vi "Auto_Step.vi"() -> ()   [LabVIEW 2020]
uses:
  Global_Variable/A180648.vi
  Global_Variable/Global.vi
panel:
  in  "判定结果":bool[][](array[boolean])=[[TRUE]]
  in  "VI引用句柄":refnum<vi>
  in  "前序OK？":string
  out "第三颗螺丝加力":bool
  out "第二颗螺丝加力":bool
  out "第一颗螺丝加力":bool
  out "磨合次数":i32
  in  "STEP":string
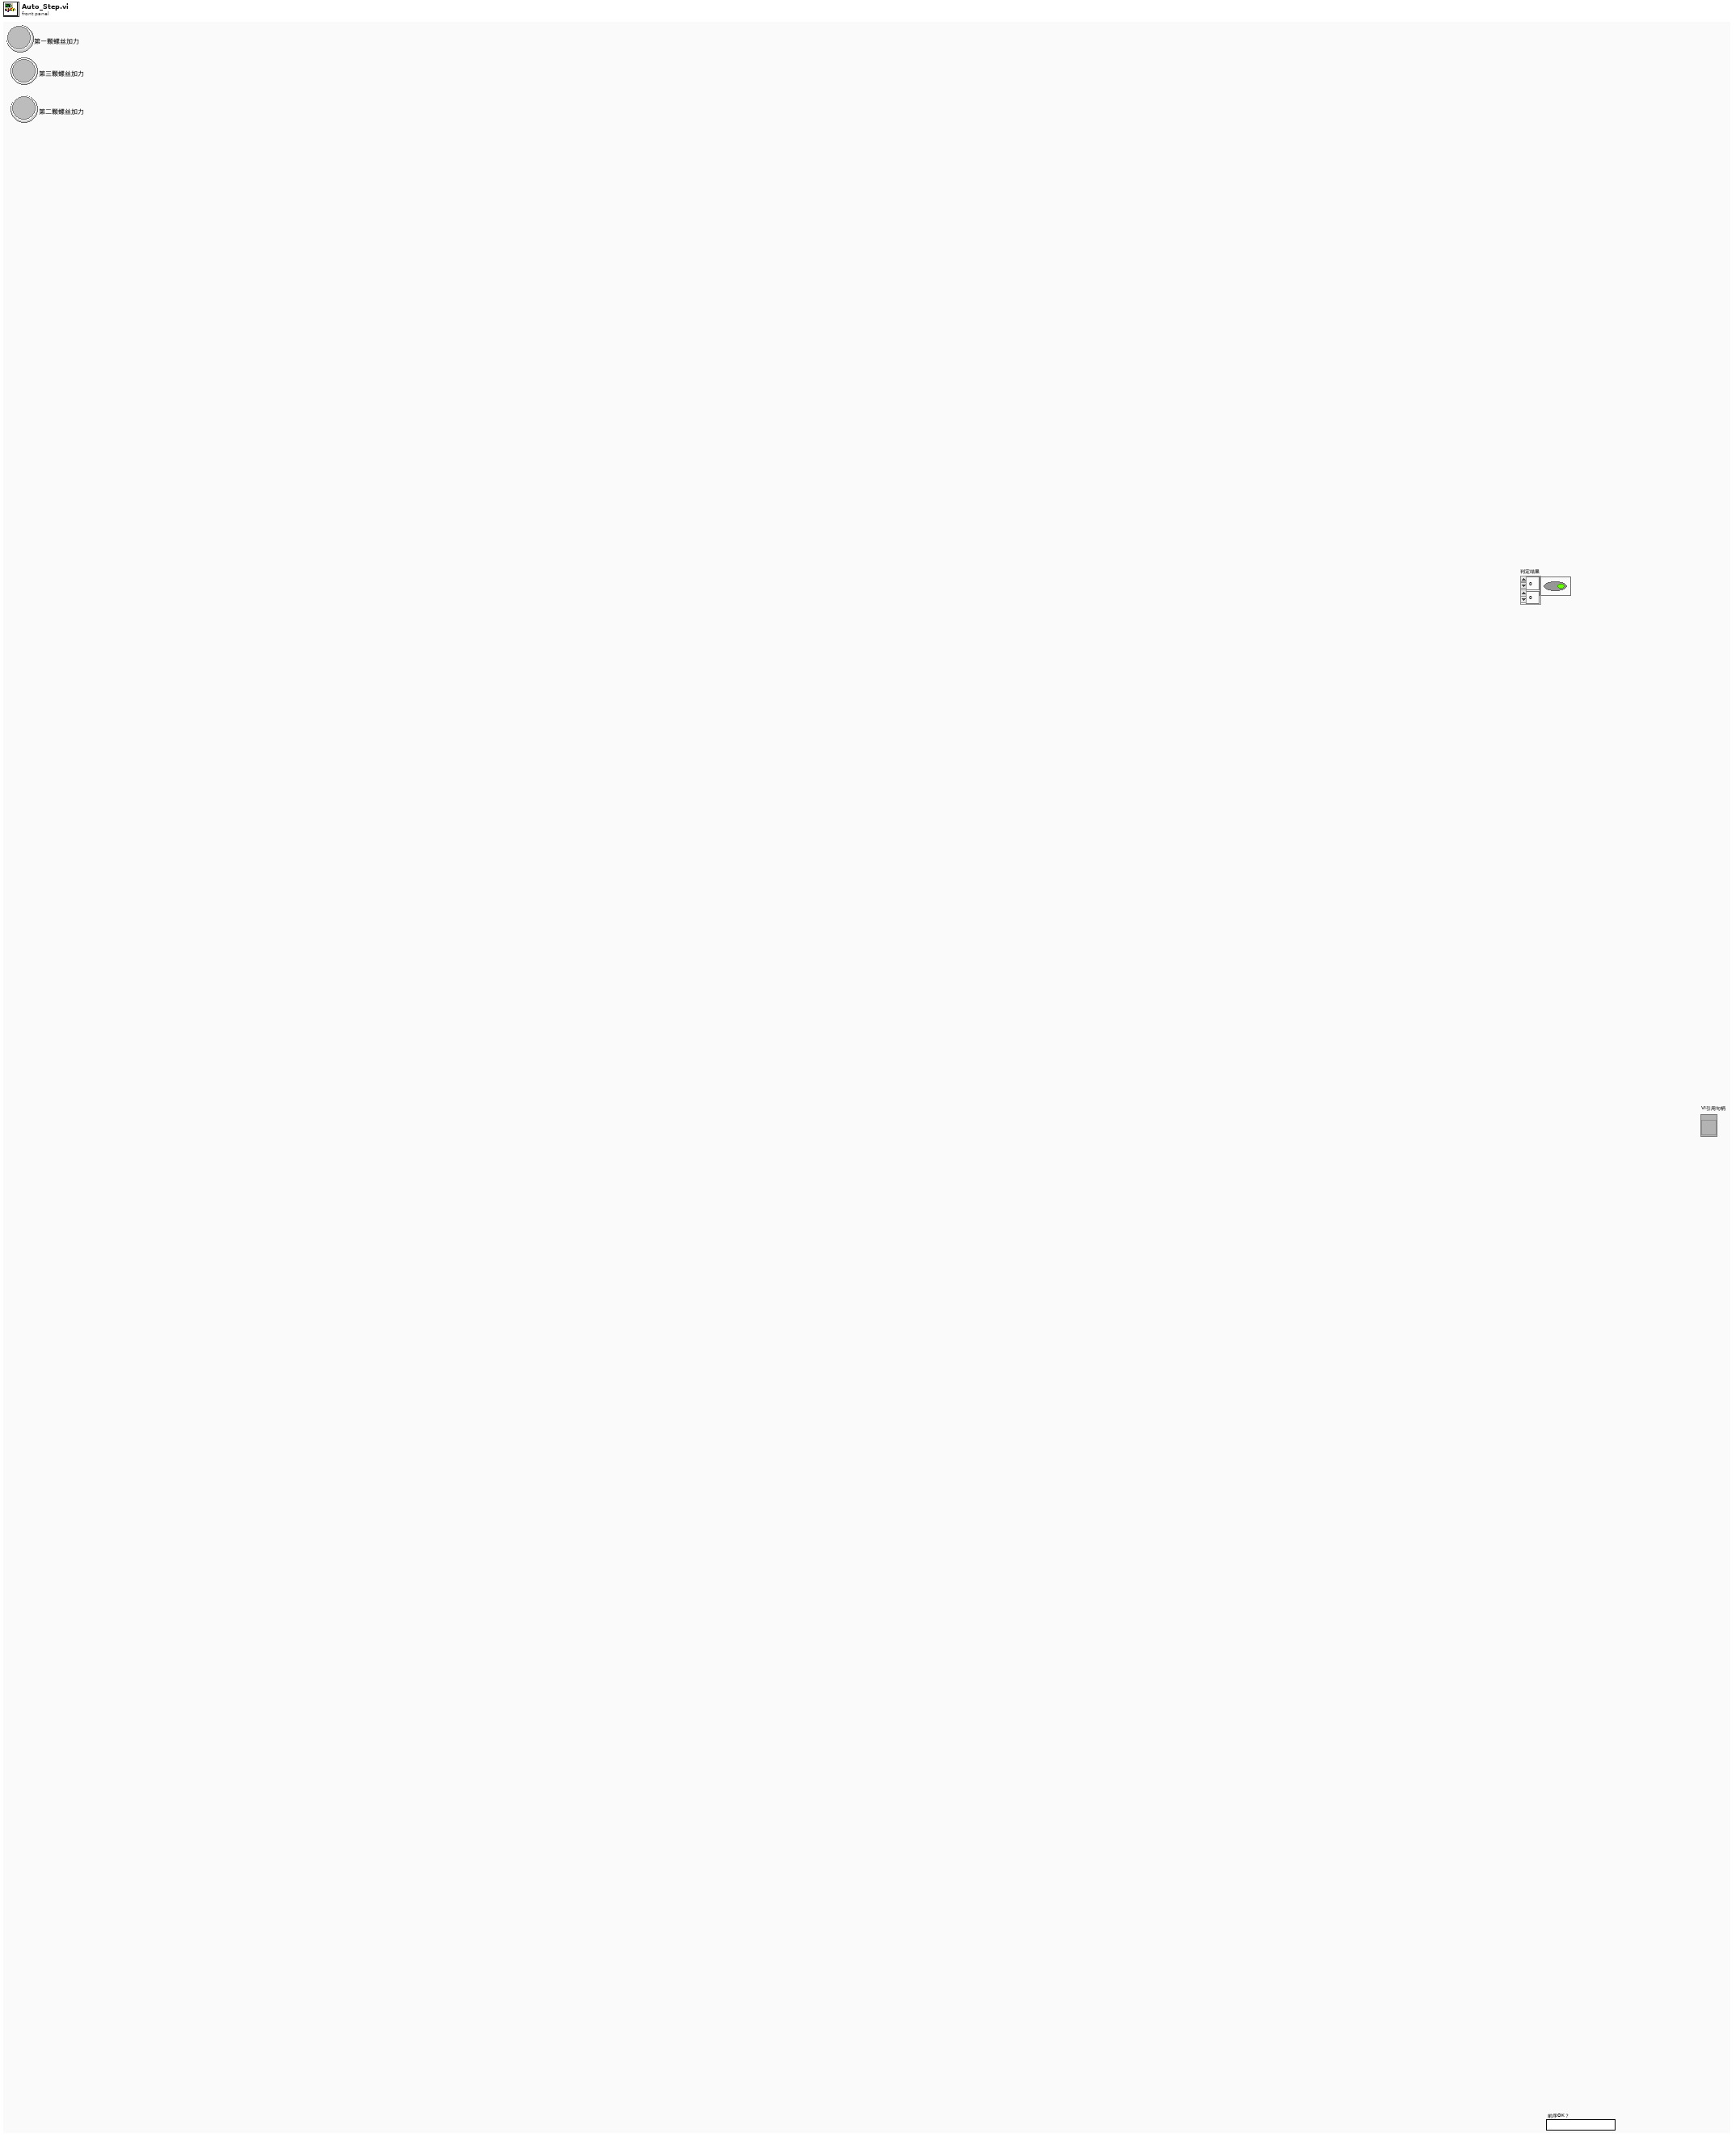
[diagram p1: front panel]
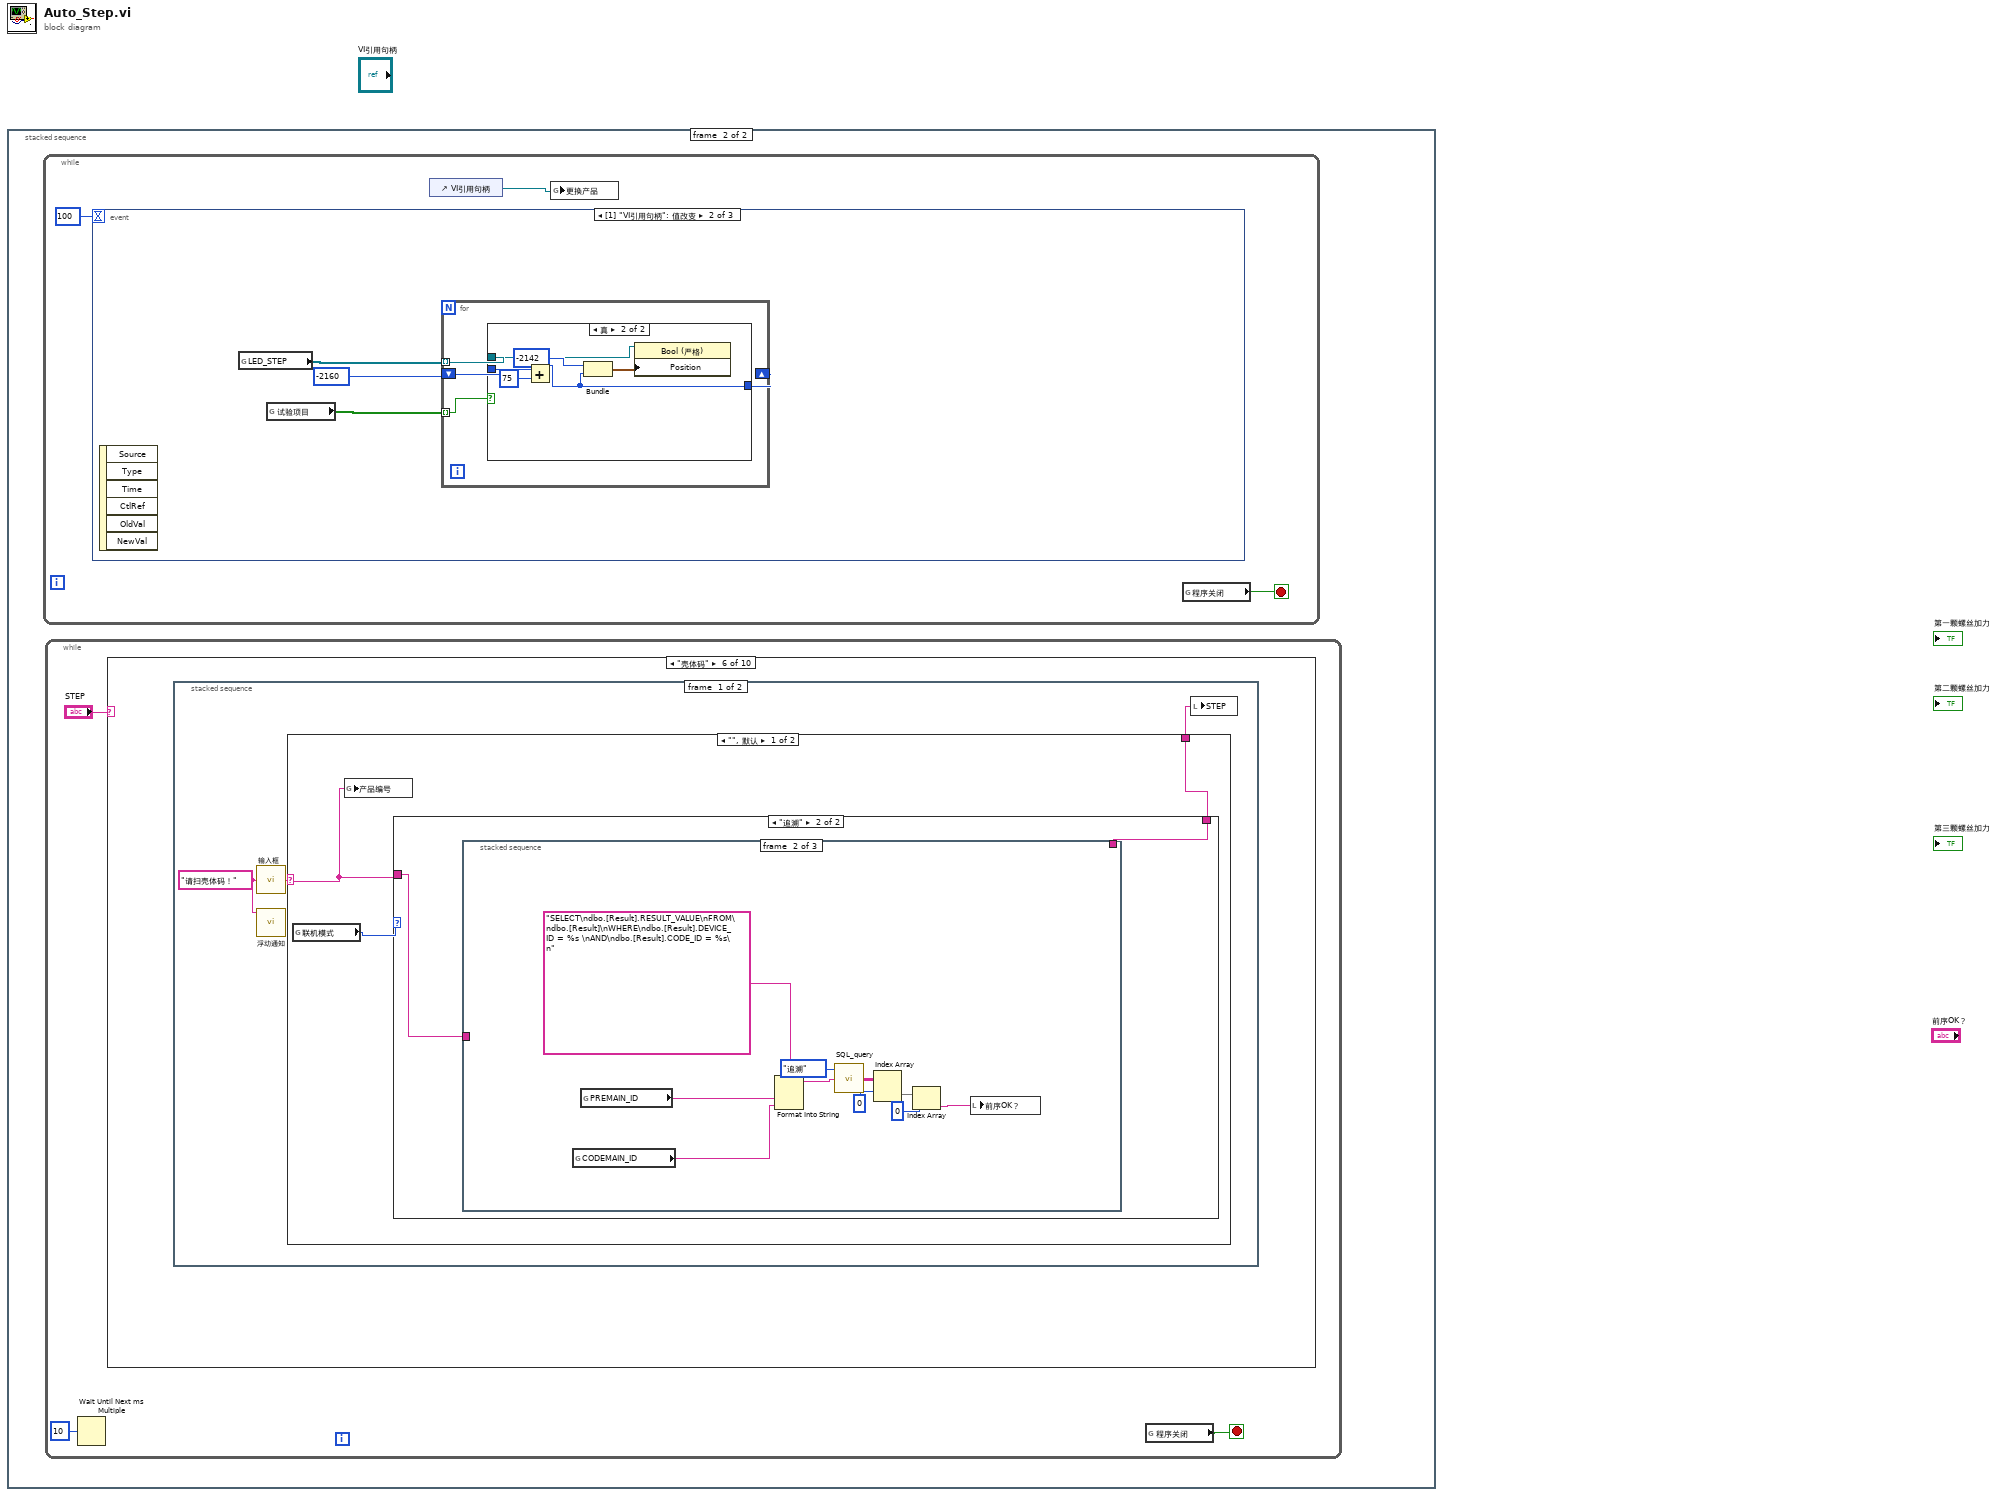
[diagram p0: block diagram]
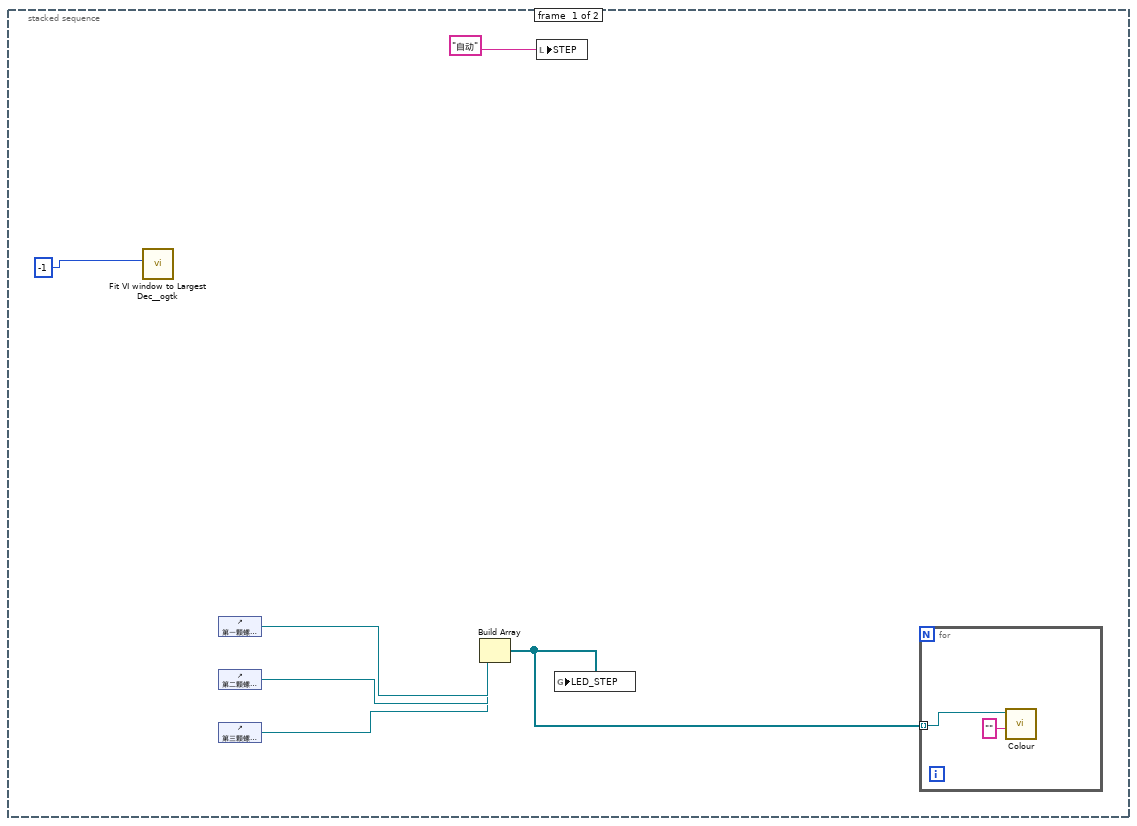
[diagram p2: hidden frame]
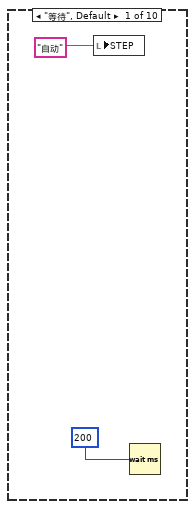
[diagram p3: hidden frame]
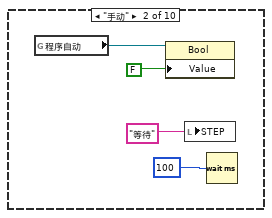
[diagram p4: hidden frame]
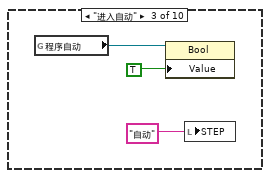
[diagram p5: hidden frame]
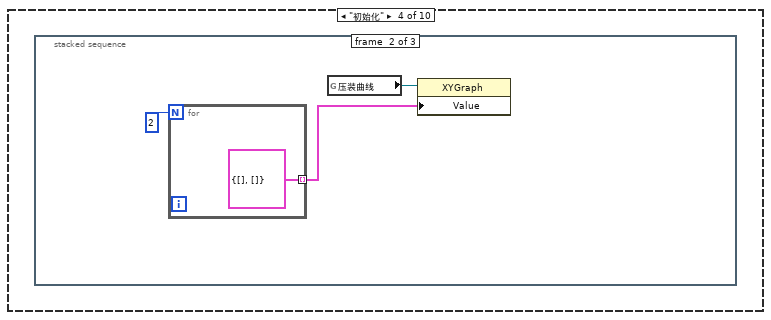
[diagram p6: hidden frame]
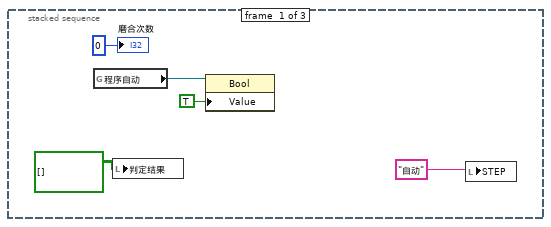
[diagram p7: hidden frame]
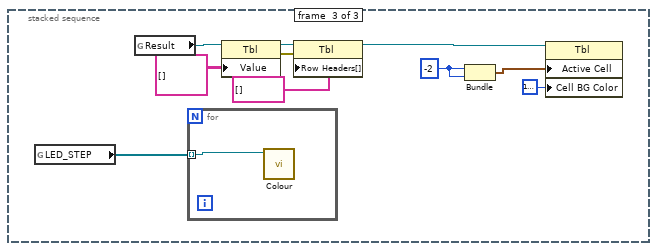
[diagram p8: hidden frame]
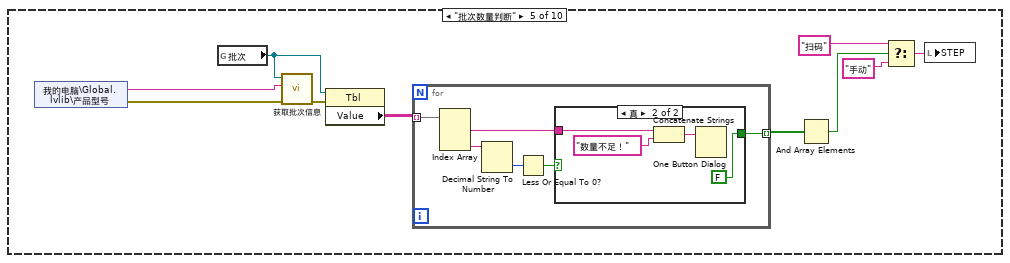
[diagram p9: hidden frame]
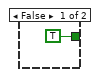
[diagram p10: hidden frame]
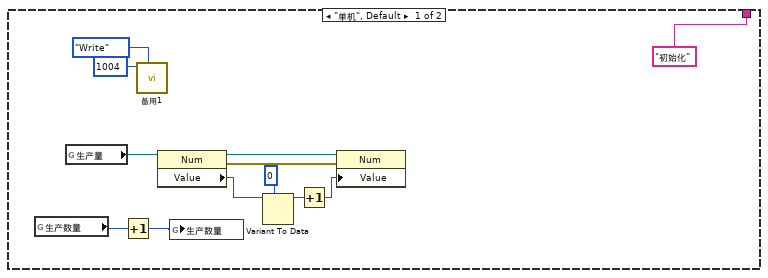
[diagram p11: hidden frame]
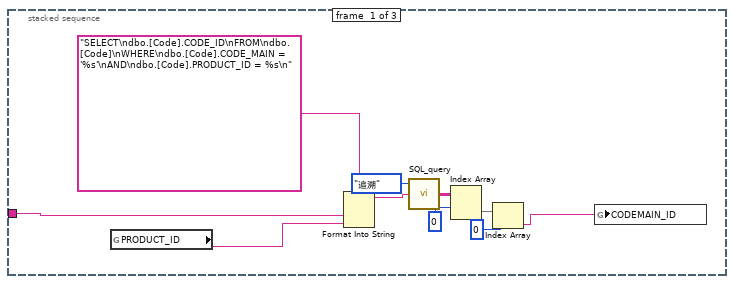
[diagram p12: hidden frame]
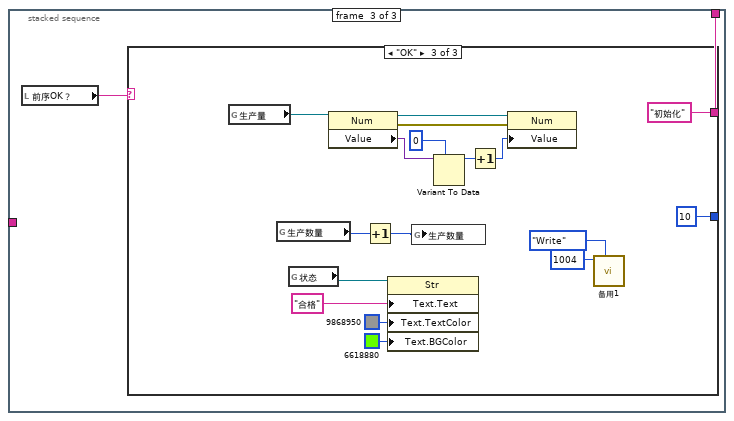
[diagram p13: hidden frame]
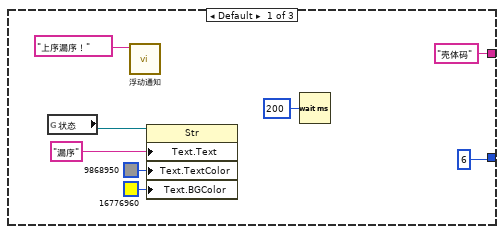
[diagram p14: hidden frame]
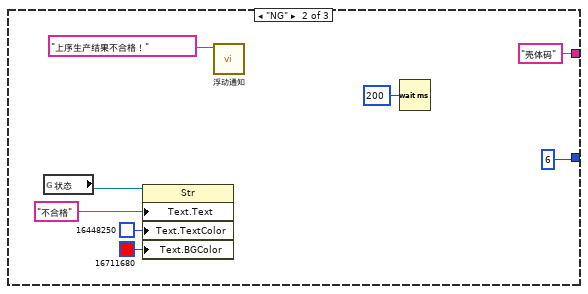
[diagram p15: hidden frame]
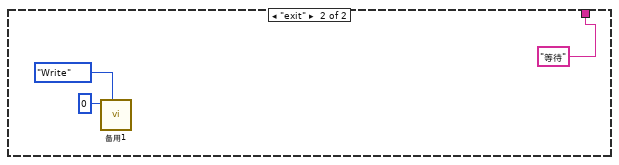
[diagram p16: hidden frame]
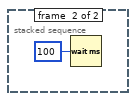
[diagram p17: hidden frame]
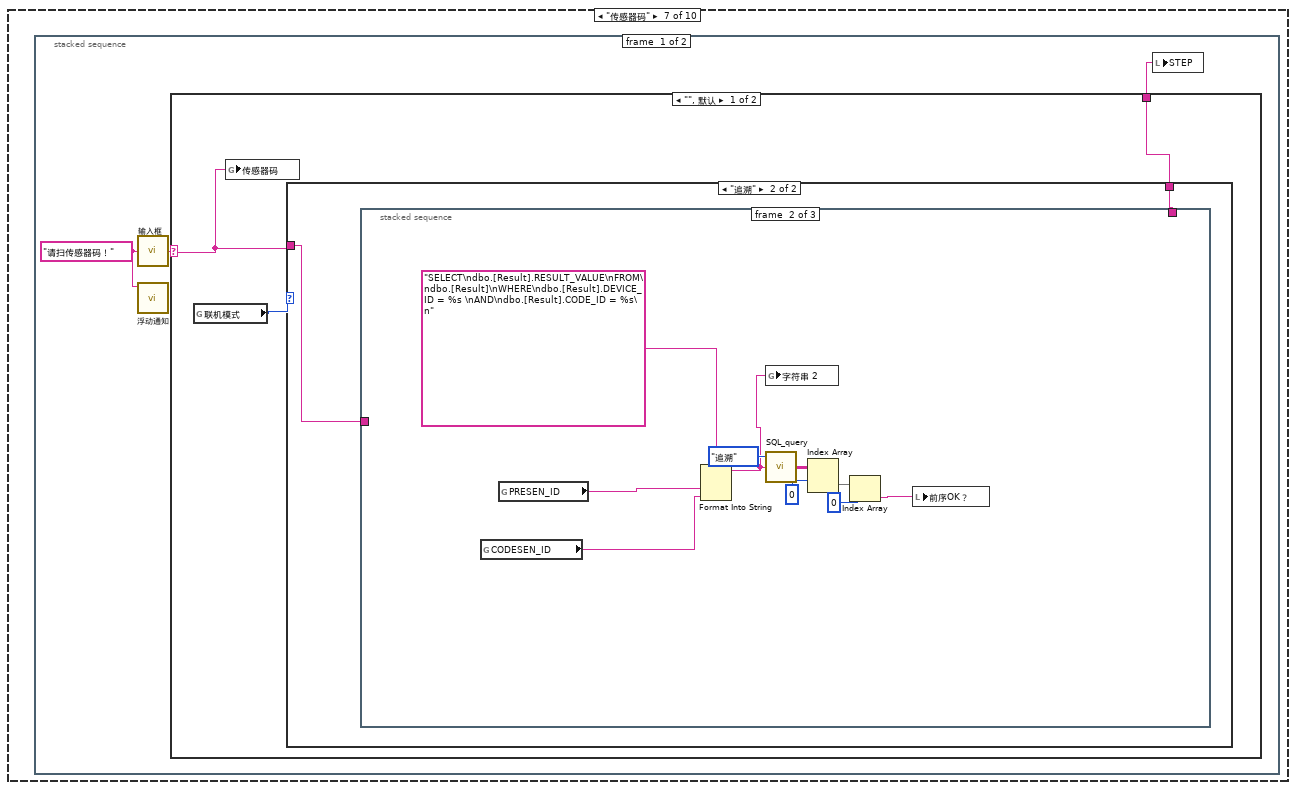
[diagram p18: hidden frame]
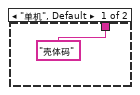
[diagram p19: hidden frame]
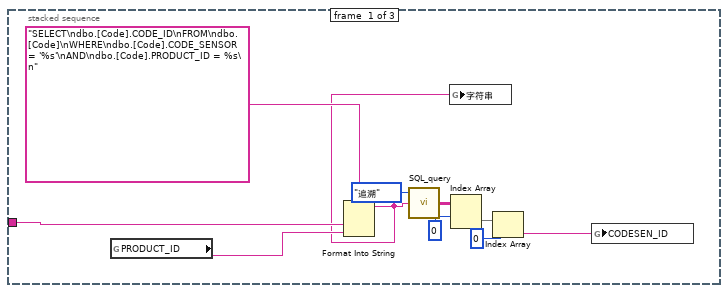
[diagram p20: hidden frame]
diagram:
  n1 = stacked-sequence {
    frame #0 {
      n2 = call <userlib>:"Fit VI window to Largest Dec__ogtk.vi"("border spacing (2 px)"=-1) -> ()  [unwired: 5 in, 2 out]
      n3 = control-ref of="第一颗螺丝加力"() -> (w4:refnum<vi>)
      n4 = control-ref of="第二颗螺丝加力"() -> (w3:refnum<vi>)
      n5 = control-ref of="第三颗螺丝加力"() -> (w2:refnum<vi>)
      n6 = Build Array(w4, w3, w2) -> (w1:refnum<vi>[])
      n7 = local write "STEP"("自动" ("STEP")) -> ()
      n8 = global write "A180648.vi" "LED_STEP"(w1) -> ()
      n9 = for {
        tunnel: w1 -> [w8] mode=indexing
        n10 = call "Colour.vi"("result"="", "colourRef"=w8) -> ()  [unwired: 9 in, 1 out]
      }
    }
    frame #1 {
      n11 = while {
        stop <- w324 stop-if-true
        n12 = event shown="[1] \"VI引用句柄\": 值改变" {
          selector: _ -> [_ _ _]
          dyn-events: _ -> [_ _ _]
          timeout: 100 -> [_ _ _]
          event Timeout {
            n13 = event-data() -> ()  [unwired: 1 in, 3 out]
          }
          event "VI引用句柄": Value Change {
            n14 = event-data() -> ()  [unwired: 1 in, 6 out]
            n15 = global read "A180648.vi" "LED_STEP"() -> (w326:refnum<vi>[])
            n16 = global read "Global.vi" "试验项目"() -> (w327:bool[])
            n17 = for "For循环" {
              tunnel: w327 -> [w329] mode=indexing
              tunnel: w326 -> [w332] mode=indexing
              shift-right: [w330] -> _
              shift-left: -2160 -> [w331]
              n18 = case shown="真" w329 {
                tunnel: w332 -> [w334 w336]
                tunnel: w331 -> [w335 w341]
                tunnel: [w335 w338] -> w330
                frame False {
                  n19 = property class="Bool (严格)"(reference=w334, "Top"=2000 ("位置:置顶")) -> ()  [unwired: 1 in, 2 out]
                }
                frame True {
                  n20 = Add(x=w341, y=75) -> (x+y=w338:i32)
                  n21 = Bundle(-2142, w338) -> (w339:cluster{i32, i32})  [unwired: 1 in]
                  n22 = property class="Bool (严格)"(reference=w336, "Position"=w339) -> ()  [unwired: 1 in, 2 out]
                }
              }
            }
          }
          event Panel Close {
            n23 = event-data() -> ()  [unwired: 1 in, 4 out]
            n24 = global write "Global.vi" "程序关闭"(TRUE ("程序关闭")) -> ()
          }
        }
        n25 = control-ref of="VI引用句柄"() -> (w323:refnum<vi>)
        n26 = global write "Global.vi" "更换产品"(w323) -> ()
        n27 = global read "Global.vi" "程序关闭"() -> (w324:bool)
      }
      n28 = while {
        stop <- w10 stop-if-true
        n29 = Wait Until Next ms Multiple(millisecond multiple=u32 10 ("毫秒倍数")) -> ()  [unwired: 1 out]
        n30 = case shown="\"壳体码\"" "STEP" {
          selector: "STEP" -> [_ _ _ _ _ _ _ w208 _ _]
          frame "等待", Default {
            n31 = local write "STEP"("自动" ("STEP")) -> ()
            n32 = Wait (ms)(milliseconds to wait=u32 200 ("等待时间（毫秒）")) -> ()  [unwired: 1 out]
          }
          frame "手动" {
            n33 = global read "Global.vi" "程序自动"() -> (w15:refnum<vi>)
            n34 = property class="Bool"(reference=w15, "Value"=FALSE) -> ()  [unwired: 1 in, 2 out]
            n35 = local write "STEP"("等待" ("STEP")) -> ()
            n36 = Wait (ms)(milliseconds to wait=u32 100 ("等待时间（毫秒）")) -> ()  [unwired: 1 out]
          }
          frame "进入自动" {
            n37 = global read "Global.vi" "程序自动"() -> (w19:refnum<vi>)
            n38 = property class="Bool"(reference=w19, "Value"=TRUE) -> ()  [unwired: 1 in, 2 out]
            n39 = local write "STEP"("自动" ("STEP")) -> ()
          }
          frame "初始化" {
            n40 = stacked-sequence {
              frame #0 {
                n41 = global read "Global.vi" "程序自动"() -> (w24:refnum<vi>)
                n42 = local write "判定结果"(bool[][] [] ("判定结果")) -> ()
                n43 = property class="Bool"(reference=w24, "Value"=TRUE) -> ()  [unwired: 1 in, 2 out]
                n44 = local write "STEP"("自动" ("result")) -> ()
                "磨合次数" <- 0 ("磨合次数")
              }
              frame #1 {
                n45 = for {
                  N: 2 -> [_]
                  tunnel: [cluster{dbl[], dbl[]} {[], []}] -> w26 mode=indexing
                }
                n46 = global read "A180648.vi" "压装曲线"() -> (w27:refnum<vi>)
                n47 = property class="XYGraph"(reference=w27, "Value"=w26) -> ()  [unwired: 1 in, 2 out]
              }
              frame #2 {
                w33 = -2
                n48 = global read "A180648.vi" "LED_STEP"() -> (w30:refnum<vi>[])
                n49 = global read "Global.vi" "Result"() -> (w37:refnum<vi>)
                n50 = for {
                  tunnel: w30 -> [w40] mode=indexing
                  n51 = call "Colour.vi"("colourRef"=w40) -> ()  [unwired: 10 in, 1 out]
                }
                n52 = property class="Tbl"(reference=w37, "Value"=string[][] []) -> (reference out=w38:refnum<vi>, error out=w39:errorcluster)  [unwired: 1 in]
                n53 = property class="Tbl"(reference=w38, error in=w39, "Row Headers[]"=string[] [] ("行首字符串[]")) -> (reference out=w34:refnum<vi>)  [unwired: 1 out]
                n54 = Bundle(w33, w33) -> (w32:cluster{i32, i32})  [unwired: 1 in]
                n55 = property class="Tbl"(reference=w34, "Active Cell"=w32, "Cell BG Color"=u32 16777216 ("活动单元格:单元格背景色")) -> ()  [unwired: 1 in, 2 out]
              }
            }
          }
          frame "批次数量判断" {
            n56 = shared-variable "我的电脑\\Global.lvlib\\产品型号"() -> (w46:string, error out=w49:errorcluster)  [unwired: 1 in]
            n57 = global read "Global.vi" "批次"() -> (w47:refnum<vi>)
            n58 = call "获取批次信息.vi"("error in (no error)"=w49, "产品型号"=w46, "Tbl引用句柄"=w47) -> ("error out"=w48:errorcluster)  [unwired: 7 in, 1 out]
            n59 = property class="Tbl"(reference=w47, error in=w48) -> ("Value"=w50:string[][])  [unwired: 2 out]
            n60 = for {
              tunnel: w50 -> [w56] mode=indexing
              tunnel: [w51] -> w45 mode=indexing
              n61 = Index Array(array=w56) -> (element #1=w52:string, element #3=w55:string)  [unwired: 3 in, 1 out]
              n62 = Decimal String To Number(string=w55) -> (number=w54:i32)  [unwired: 2 in, 1 out]
              n63 = Less Or Equal To 0?(x=w54) -> (x <= 0?=w53:bool)
              n64 = case shown="真" w53 {
                tunnel: w52 -> [_ w61]
                tunnel: [TRUE FALSE] -> w51
                frame False {
                }
                frame True {
                  n65 = Concatenate Strings(w61, "数量不足！" ("字符串")) -> (w59:string)
                  n66 = One Button Dialog(message=w59) -> ()  [unwired: 1 in, 1 out]
                }
              }
            }
            n67 = And Array Elements(Boolean array=w45) -> (logical AND=w44:bool)
            n68 = Select(t="扫码" ("STEP"), s=w44, f="手动" ("STEP")) -> (s? t:f=w41:string)
            n69 = local write "STEP"(w41) -> ()
          }
          frame "壳体码" {
            n70 = stacked-sequence {
              frame #0 {
                w63 = "请扫壳体码！" ("提示信息")
                n71 = call "输入框.vi"("提示信息"=w63) -> ("条形码输出"=w64:string)
                n72 = call "浮动通知.vi"("通知内容"=w63) -> ()  [unwired: 11 in]
                n73 = case shown="\"\", 默认" w64 {
                  selector: w64 -> [w65 _]
                  tunnel: [w67 "等待"] -> w62
                  frame "", Default {
                    n74 = global read "Global.vi" "联机模式"() -> (w66:enum16{"单机", "追溯"})
                    n75 = global write "Global.vi" "产品编号"(w65) -> ()
                    n76 = case shown="\"追溯\"" w66 {
                      tunnel: w65 -> [_ w80]
                      tunnel: ["初始化" w81] -> w67
                      frame "单机", Default {
                        n77 = global read "Global.vi" "生产数量"() -> (w69:i32)
                        n78 = global read "Global.vi" "生产量"() -> (w72:refnum<vi>)
                        n79 = Increment(x=w69) -> (x+1=w68:i32)
                        n80 = call "备用1.vi"("枚举"=enum16{"Read", "Write"}."Write", "Status_Write"=i16 1004) -> ()  [unwired: 9 in, 1 out]
                        n81 = property class="Num"(reference=w72) -> (reference out=w75:refnum<vi>, error out=w76:errorcluster, "Value"=w77:variant)  [unwired: 1 in]
                        n82 = global write "Global.vi" "生产数量"(w68) -> ()
                        n83 = Variant To Data(type=u32 0, Variant=w77) -> (data=w78:u32)  [unwired: 1 in, 1 out]
                        n84 = Increment(x=w78) -> (x+1=w79:u32)
                        n85 = property class="Num"(reference=w75, error in=w76, "Value"=w79) -> ()  [unwired: 2 out]
                      }
                      frame "追溯" {
                        n86 = stacked-sequence {
                          tunnel: w80 -> [w89 _ _]
                          tunnel: [_ _ w103] -> w81
                          frame #0 {
                            n87 = global read "追溯Global.vi" "PRODUCT_ID"() -> (w83:string)
                            n88 = Format Into String(format string="SELECT\ndbo.[Code].CODE_ID\nFROM\ndbo.[Code]\nWHERE\ndbo.[Code].CODE_MAIN = '%s'\nAND\ndbo.[Code].PRODUCT_ID = %s\n" ("格式字符串"), w89, w83) -> (resulting string=w88:string)  [unwired: 2 in, 1 out]
                            n89 = call "SQL_query.vi"("SQL query"=w88, "联机模式"=enum16{"单机", "追溯"}."追溯") -> ("data"=w91:string[][])  [unwired: 2 in, 1 out]
                            n90 = Index Array(array=w91, index (row)=0 ("索引 (行)")) -> (element=w90:string[])  [unwired: 1 in]
                            n91 = Index Array(array=w90, index=0 ("索引")) -> (element=w84:string)
                            n92 = global write "追溯Global.vi" "CODEMAIN_ID"(w84) -> ()
                          }
                          frame #1 {
                            n93 = global read "追溯Global.vi" "CODEMAIN_ID"() -> (w92:string)
                            n94 = global read "追溯Global.vi" "PREMAIN_ID"() -> (w94:string)
                            n95 = Format Into String(format string="SELECT\ndbo.[Result].RESULT_VALUE\nFROM\ndbo.[Result]\nWHERE\ndbo.[Result].DEVICE_ID = %s \nAND\ndbo.[Result].CODE_ID = %s\n" ("格式字符串"), w94, w92) -> (resulting string=w99:string)  [unwired: 2 in, 1 out]
                            n96 = call "SQL_query.vi"("SQL query"=w99, "联机模式"=enum16{"单机", "追溯"}."追溯") -> ("data"=w101:string[][])  [unwired: 2 in, 1 out]
                            n97 = Index Array(array=w101, index (row)=0 ("索引 (行)")) -> (element=w100:string[])  [unwired: 1 in]
                            n98 = Index Array(array=w100, index=0 ("索引")) -> (element=w95:string)
                            n99 = local write "前序OK？"(w95) -> ()
                          }
                          frame #2 {
                            n100 = local read "前序OK？"() -> (w102:string)
                            n101 = case shown="\"OK\"" w102 {
                              tunnel: [i16 6 ("设备状态控制字") i16 6 ("设备状态控制字") i16 10 ("设备状态控制字")] -> _
                              tunnel: ["壳体码" "壳体码" "初始化"] -> w103
                              frame Default {
                                n102 = global read "Global.vi" "状态"() -> (w107:refnum<vi>)
                                n103 = call "浮动通知.vi"("通知内容"="上序漏序！" ("Status")) -> ()  [unwired: 11 in]
                                n104 = property class="Str"(reference=w107, "Text.Text"="漏序" ("文本.文本"), "Text.TextColor"=u32 9868950 ("文本.文本颜色:文本颜色"), "Text.BGColor"=u32 16776960 ("文本.文本颜色:背景色")) -> ()  [unwired: 1 in, 2 out]
                                n105 = Wait (ms)(milliseconds to wait=u32 200 ("等待时间（毫秒）")) -> ()  [unwired: 1 out]
                              }
                              frame "NG" {
                                n106 = global read "Global.vi" "状态"() -> (w115:refnum<vi>)
                                n107 = property class="Str"(reference=w115, "Text.Text"="不合格" ("文本.文本"), "Text.TextColor"=u32 16448250 ("文本.文本颜色:文本颜色"), "Text.BGColor"=u32 16711680 ("文本.文本颜色:背景色")) -> ()  [unwired: 1 in, 2 out]
                                n108 = call "浮动通知.vi"("通知内容"="上序生产结果不合格！" ("Status")) -> ()  [unwired: 11 in]
                                n109 = Wait (ms)(milliseconds to wait=u32 200 ("等待时间（毫秒）")) -> ()  [unwired: 1 out]
                              }
                              frame "OK" {
                                n110 = global read "Global.vi" "生产量"() -> (w128:refnum<vi>)
                                n111 = global read "Global.vi" "生产数量"() -> (w123:i32)
                                n112 = global read "Global.vi" "状态"() -> (w127:refnum<vi>)
                                n113 = property class="Num"(reference=w128) -> (reference out=w135:refnum<vi>, error out=w134:errorcluster, "Value"=w133:variant)  [unwired: 1 in]
                                n114 = Increment(x=w123) -> (x+1=w122:i32)
                                n115 = property class="Str"(reference=w127, "Text.Text"="合格" ("文本.文本"), "Text.TextColor"=u32 9868950 ("文本.文本颜色:文本颜色"), "Text.BGColor"=u32 6618880 ("文本.文本颜色:背景色")) -> ()  [unwired: 1 in, 2 out]
                                n116 = global write "Global.vi" "生产数量"(w122) -> ()
                                n117 = Variant To Data(type=u32 0, Variant=w133) -> (data=w132:u32)  [unwired: 1 in, 1 out]
                                n118 = Increment(x=w132) -> (x+1=w131:u32)
                                n119 = property class="Num"(reference=w135, error in=w134, "Value"=w131) -> ()  [unwired: 2 out]
                                n120 = call "备用1.vi"("枚举"=enum16{"Read", "Write"}."Write", "Status_Write"=i16 1004) -> ()  [unwired: 9 in, 1 out]
                              }
                            }
                          }
                        }
                      }
                    }
                  }
                  frame "exit" {
                    n121 = call "备用1.vi"("枚举"=enum16{"Read", "Write"}."Write", "Status_Write"=i16 0) -> ()  [unwired: 9 in, 1 out]
                  }
                }
                n122 = local write "STEP"(w62) -> ()
              }
              frame #1 {
                n123 = Wait (ms)(milliseconds to wait=u32 100 ("等待时间（毫秒）")) -> ()  [unwired: 1 out]
              }
            }
          }
          frame "传感器码" {
            n124 = stacked-sequence {
              frame #0 {
                w142 = "请扫传感器码！" ("提示信息")
                n125 = call "输入框.vi"("提示信息"=w142) -> ("条形码输出"=w143:string)
                n126 = call "浮动通知.vi"("通知内容"=w142) -> ()  [unwired: 11 in]
                n127 = case shown="\"\", 默认" w143 {
                  selector: w143 -> [w144 _]
                  tunnel: [w146 "等待"] -> w141
                  frame "", Default {
                    n128 = global read "Global.vi" "联机模式"() -> (w145:enum16{"单机", "追溯"})
                    n129 = global write "Global.vi" "传感器码"(w144) -> ()
                    n130 = case shown="\"追溯\"" w145 {
                      tunnel: w144 -> [_ w148]
                      tunnel: ["壳体码" w149] -> w146
                      frame "单机", Default {
                      }
                      frame "追溯" {
                        n131 = stacked-sequence {
                          tunnel: w148 -> [w157 _ _]
                          tunnel: [_ _ w171] -> w149
                          frame #0 {
                            n132 = global read "追溯Global.vi" "PRODUCT_ID"() -> (w152:string)
                            n133 = Format Into String(format string="SELECT\ndbo.[Code].CODE_ID\nFROM\ndbo.[Code]\nWHERE\ndbo.[Code].CODE_SENSOR = '%s'\nAND\ndbo.[Code].PRODUCT_ID = %s\n" ("格式字符串"), w157, w152) -> (resulting string=w150:string)  [unwired: 2 in, 1 out]
                            n134 = call "SQL_query.vi"("SQL query"=w150, "联机模式"=enum16{"单机", "追溯"}."追溯") -> ("data"=w159:string[][])  [unwired: 2 in, 1 out]
                            n135 = global write "追溯Global.vi" "字符串"(w150) -> ()
                            n136 = Index Array(array=w159, index (row)=0 ("索引 (行)")) -> (element=w158:string[])  [unwired: 1 in]
                            n137 = Index Array(array=w158, index=0 ("索引")) -> (element=w153:string)
                            n138 = global write "追溯Global.vi" "CODESEN_ID"(w153) -> ()
                          }
                          frame #1 {
                            n139 = global read "追溯Global.vi" "CODESEN_ID"() -> (w160:string)
                            n140 = global read "追溯Global.vi" "PRESEN_ID"() -> (w162:string)
                            n141 = Format Into String(format string="SELECT\ndbo.[Result].RESULT_VALUE\nFROM\ndbo.[Result]\nWHERE\ndbo.[Result].DEVICE_ID = %s \nAND\ndbo.[Result].CODE_ID = %s\n" ("格式字符串"), w162, w160) -> (resulting string=w161:string)  [unwired: 2 in, 1 out]
                            n142 = global write "追溯Global.vi" "字符串 2"(w161) -> ()
                            n143 = call "SQL_query.vi"("SQL query"=w161, "联机模式"=enum16{"单机", "追溯"}."追溯") -> ("data"=w169:string[][])  [unwired: 2 in, 1 out]
                            n144 = Index Array(array=w169, index (row)=0 ("索引 (行)")) -> (element=w168:string[])  [unwired: 1 in]
                            n145 = Index Array(array=w168, index=0 ("索引")) -> (element=w164:string)
                            n146 = local write "前序OK？"(w164) -> ()
                          }
                          frame #2 {
                            n147 = local read "前序OK？"() -> (w170:string)
                            n148 = case shown="\"NG\"" w170 {
                              tunnel: [i16 6 ("设备状态控制字") i16 6 ("设备状态控制字") i16 10 ("设备状态控制字")] -> _
                              tunnel: ["传感器码" "传感器码" "壳体码"] -> w171
                              frame Default {
                                n149 = global read "Global.vi" "状态"() -> (w175:refnum<vi>)
                                n150 = property class="Str"(reference=w175, "Text.Text"="漏序" ("文本.文本"), "Text.TextColor"=u32 9868950 ("文本.文本颜色:文本颜色"), "Text.BGColor"=u32 16776960 ("文本.文本颜色:背景色")) -> ()  [unwired: 1 in, 2 out]
                                n151 = call "浮动通知.vi"("通知内容"="上序漏序！" ("Status")) -> ()  [unwired: 11 in]
                                n152 = Wait (ms)(milliseconds to wait=u32 200 ("等待时间（毫秒）")) -> ()  [unwired: 1 out]
                              }
                              frame "NG" {
                                n153 = global read "Global.vi" "状态"() -> (w183:refnum<vi>)
                                n154 = property class="Str"(reference=w183, "Text.Text"="不合格" ("文本.文本"), "Text.TextColor"=u32 16448250 ("文本.文本颜色:文本颜色"), "Text.BGColor"=u32 16711680 ("文本.文本颜色:背景色")) -> ()  [unwired: 1 in, 2 out]
                                n155 = call "浮动通知.vi"("通知内容"="上序生产结果不合格！" ("Status")) -> ()  [unwired: 11 in]
                                n156 = Wait (ms)(milliseconds to wait=u32 200 ("等待时间（毫秒）")) -> ()  [unwired: 1 out]
                              }
                              frame "OK" {
                                n157 = global read "Global.vi" "生产量"() -> (w192:refnum<vi>)
                                n158 = global read "Global.vi" "状态"() -> (w191:refnum<vi>)
                                n159 = property class="Num"(reference=w192) -> (reference out=w199:refnum<vi>, error out=w198:errorcluster, "Value"=w197:variant)  [unwired: 1 in]
                                n160 = property class="Str"(reference=w191, "Text.Text"="合格" ("文本.文本"), "Text.TextColor"=u32 9868950 ("文本.文本颜色:文本颜色"), "Text.BGColor"=u32 6618880 ("文本.文本颜色:背景色")) -> ()  [unwired: 1 in, 2 out]
                                n161 = Variant To Data(type=u32 0, Variant=w197) -> (data=w196:u32)  [unwired: 1 in, 1 out]
                                n162 = Increment(x=w196) -> (x+1=w195:u32)
                                n163 = property class="Num"(reference=w199, error in=w198, "Value"=w195) -> ()  [unwired: 2 out]
                              }
                            }
                          }
                        }
                      }
                    }
                  }
                  frame "exit" {
                    n164 = call "备用1.vi"("枚举"=enum16{"Read", "Write"}."Write", "Status_Write"=i16 0) -> ()  [unwired: 9 in, 1 out]
                  }
                }
                n165 = local write "STEP"(w141) -> ()
              }
              frame #1 {
                n166 = Wait (ms)(milliseconds to wait=u32 100 ("等待时间（毫秒）")) -> ()  [unwired: 1 out]
              }
            }
          }
          frame "自动" {
            n167 = global read "A180648.vi" "LED_STEP"() -> (w207:refnum<vi>[])
            n168 = global read "Global.vi" "设备状态"() -> (w206:i16)
            n169 = case shown="71" w206 {
              tunnel: w207 -> [_ _ _ w217 w223 w230 w235 w236 _ _ _ w239 w243 w248 w253 w258 w264 _ w269 _ _ _ _]
              tunnel: w208 -> [_ _ _ _ _ _ _ _ _ _ _ _ _ _ _ _ _ _ _ _ _ _ _]
              frame Default {
              }
              frame -128 {
                n170 = call "浮动通知.vi"("通知内容"="复位中……" ("Status")) -> ()  [unwired: 11 in]
                n171 = global read "Global.vi" "程序自动"() -> (w212:refnum<vi>)
                n172 = property class="Bool"(reference=w212, "Value"=FALSE) -> ()  [unwired: 1 in, 2 out]
              }
              frame 0 {
              }
              frame 2 {
                n173 = Index Array(array=w217) -> (element=w216:refnum<vi>)  [unwired: 1 in]
                n174 = call "浮动通知.vi"("通知内容"="请拧紧第一颗螺丝" ("Status")) -> ()  [unwired: 11 in]
                n175 = call "Colour.vi"("result"="等待", "colourRef"=w216) -> ()  [unwired: 9 in, 1 out]
              }
              frame 3 {
                n176 = Index Array(array=w223) -> (element #1=w222:refnum<vi>, element #2=w218:refnum<vi>)  [unwired: 2 in]
                n177 = call "浮动通知.vi"("通知内容"="请拧紧第二颗螺丝" ("Status")) -> ()  [unwired: 11 in]
                n178 = call "Colour.vi"("result"="等待", "colourRef"=w218) -> ()  [unwired: 9 in, 1 out]
                n179 = call "Colour.vi"("result"="OK", "colourRef"=w222) -> ()  [unwired: 9 in, 1 out]
              }
              frame 4 {
                n180 = Index Array(array=w230, index #1=1 ("索引")) -> (element #1=w229:refnum<vi>, element #2=w225:refnum<vi>)  [unwired: 1 in]
                n181 = call "浮动通知.vi"("通知内容"="请拧紧第三颗螺丝" ("Status")) -> ()  [unwired: 11 in]
                n182 = call "Colour.vi"("result"="等待", "colourRef"=w225) -> ()  [unwired: 9 in, 1 out]
                n183 = call "Colour.vi"("result"="OK", "colourRef"=w229) -> ()  [unwired: 9 in, 1 out]
              }
              frame 5 {
                n184 = Index Array(array=w235, index #1=2 ("索引")) -> (element #1=w234:refnum<vi>)  [unwired: 1 in, 1 out]
                n185 = call "浮动通知.vi"("通知内容"="请标记" ("Status")) -> ()  [unwired: 11 in]
                n186 = call "Colour.vi"("result"="OK", "colourRef"=w234) -> ()  [unwired: 9 in, 1 out]
              }
              frame 6 {
                n187 = Index Array(array=w236, index=0 ("索引")) -> ()  [unwired: 1 out]
              }
              frame 7 {
              }
              frame 8 {
              }
              frame 9 {
              }
              frame 10 {
                n188 = Index Array(array=w239, index #1=0 ("索引")) -> ()  [unwired: 1 in, 2 out]
                n189 = call "Colour.vi"("result"="OK") -> ()  [unwired: 10 in, 1 out]
                n190 = call "Colour.vi"("result"="等待") -> ()  [unwired: 10 in, 1 out]
                n191 = call "浮动通知.vi"("通知内容"="请安装下轴螺栓并确认扭矩！" ("Status")) -> ()  [unwired: 11 in]
              }
              frame 22 {
                n192 = Index Array(array=w243, index #1=1 ("索引")) -> ()  [unwired: 1 in, 2 out]
                n193 = call "浮动通知.vi"("通知内容"="请涂下轴固定螺栓色标！" ("Status")) -> ()  [unwired: 11 in]
                n194 = call "Colour.vi"("result"="OK") -> ()  [unwired: 10 in, 1 out]
                n195 = call "Colour.vi"("result"="等待") -> ()  [unwired: 10 in, 1 out]
              }
              frame 42 {
                n196 = Index Array(array=w248, index #1=3 ("索引")) -> ()  [unwired: 1 in, 2 out]
                n197 = call "浮动通知.vi"("通知内容"="请向左转动两圈！" ("Status")) -> ()  [unwired: 11 in]
                n198 = call "Colour.vi"("result"="OK") -> ()  [unwired: 10 in, 1 out]
                n199 = call "Colour.vi"("result"="等待") -> ()  [unwired: 10 in, 1 out]
              }
              frame 52 {
                n200 = Index Array(array=w253, index #1=4 ("索引")) -> ()  [unwired: 1 in, 2 out]
                n201 = call "浮动通知.vi"("通知内容"="请向右转动两圈！" ("Status")) -> ()  [unwired: 11 in]
                n202 = call "Colour.vi"("result"="OK") -> ()  [unwired: 10 in, 1 out]
                n203 = call "Colour.vi"("result"="等待") -> ()  [unwired: 10 in, 1 out]
              }
              frame 62 {
                n204 = Index Array(array=w258, index #1=5 ("索引")) -> ()  [unwired: 1 in, 2 out]
                n205 = call "Colour.vi"("result"="等待") -> ()  [unwired: 10 in, 1 out]
                n206 = call "Colour.vi"("result"="OK") -> ()  [unwired: 10 in, 1 out]
                n207 = call "浮动通知.vi"("通知内容"="请判断是否合格！" ("Status")) -> ()  [unwired: 11 in]
              }
              frame 71 {
                n208 = Index Array(array=w264, index #1=7 ("索引")) -> ()  [unwired: 1 in, 2 out]
                n209 = call "Colour.vi"("result"="等待") -> ()  [unwired: 10 in, 1 out]
                n210 = call "浮动通知.vi"("通知内容"="拆掉下传动轴辅具，安装下传动轴！" ("Status")) -> ()  [unwired: 11 in]
              }
              frame 101 {
                n211 = call "浮动通知.vi"("通知内容"="请放回检具10！" ("Status")) -> ()  [unwired: 11 in]
              }
              frame 201 {
                n212 = Index Array(array=w269, index #1=6 ("索引")) -> ()  [unwired: 1 in, 2 out]
                n213 = call "Colour.vi"("result"="NG") -> ()  [unwired: 10 in, 1 out]
                n214 = call "Colour.vi"("result"="等待") -> ()  [unwired: 10 in, 1 out]
                n215 = call "浮动通知.vi"("通知内容"="产品不合格！" ("Status")) -> ()  [unwired: 11 in]
              }
              frame 1024 {
                n216 = call "浮动通知.vi"("通知内容"="急停！" ("Status")) -> ()  [unwired: 11 in]
                n217 = global read "Global.vi" "程序自动"() -> (w274:refnum<vi>)
                n218 = property class="Bool"(reference=w274, "Value"=FALSE) -> ()  [unwired: 1 in, 2 out]
              }
              frame 3721 {
                n219 = local write "STEP"("不合格锁定" ("STEP")) -> ()
                n220 = call "浮动通知.vi"("通知内容"="产品不合格程序锁定！" ("Status")) -> ()  [unwired: 11 in]
              }
              frame 3722 {
                n221 = global read "Global.vi" "程序自动"() -> (w279:refnum<vi>)
                n222 = call "浮动通知.vi"("通知内容"="授权成功，请复位！" ("Status")) -> ()  [unwired: 11 in]
                n223 = property class="Bool"(reference=w279, "Value"=FALSE) -> ()  [unwired: 1 in, 2 out]
              }
              frame 3723 {
                n224 = call "浮动通知.vi"("通知内容"="请取出不合格产品并摆放至不合格品区！" ("Status")) -> ()  [unwired: 11 in]
              }
            }
            n225 = call "备用1.vi"() -> ("Status_Read"=w205:i16)  [unwired: 11 in]
            n226 = case shown="20" w205 {
              frame 0, Default {
              }
              frame 20 {
                n227 = local write "STEP"("判定" ("STEP")) -> ()
              }
              frame 13 {
              }
              frame 1000 {
                n228 = local write "STEP"("传感器码" ("STEP")) -> ()
              }
            }
          }
          frame "判定" {
            n229 = stacked-sequence {
              frame #0 {
                n230 = global read "Global.vi" "复测"() -> (w282:bool)
                n231 = case shown="真" w282 {
                  frame False {
                    n232 = local write "判定结果"(bool[][] [[TRUE, TRUE]] ("判定结果")) -> ()
                  }
                  frame True {
                  }
                }
              }
              frame #1 {
                n233 = local write "STEP"("报表" ("STEP")) -> ()
                n234 = call "备用1.vi"("枚举"=enum16{"Read", "Write"}."Write", "Status_Write"=i16 0) -> ()  [unwired: 9 in, 1 out]
              }
            }
          }
          frame "报表" {
            n235 = stacked-sequence {
              seq-local: [_ w290 _ _ _] -> [_ _ w295 _ _]
              frame #0 {
                n236 = global write "Global.vi" "计时开始"(FALSE ("计时开始")) -> ()
                n237 = disable-structure shown="禁用" {
                  frame Disabled {
                    n238 = global read "Global.vi" "产品编号"() -> (w289:string)
                    n239 = call "Get_CODE_ID.vi"("CODE_MAIN"=w289) -> ("CODE_ID"=w288:string)  [unwired: 10 in]
                    n240 = global write "追溯Global.vi" "CODE_ID"(w288) -> ()
                  }
                  frame Enabled {
                  }
                }
              }
              frame #1 {
                n241 = global read "Global.vi" "产品编号"() -> (w291:string)
                n242 = call "Report.vi"("文件重命名"=TRUE, "文件名称"=w291, "检测结果"="判定结果") -> ("PRODUCT_VAULE"=w290:string)  [unwired: 7 in, 1 out]
              }
              frame #2 {
                n243 = global read "Global.vi" "联机模式"() -> (w294:enum16{"单机", "追溯"})
                n244 = case shown="\"追溯\"" w294 {
                  tunnel: w295 -> [_ w297]
                  frame "单机", Default {
                  }
                  frame "追溯" {
                    n245 = global read "Global.vi" "Result"() -> (w301:refnum<vi>)
                    n246 = property class="Tbl"(reference=w301) -> (reference out=w306:refnum<vi>, error out=w303:errorcluster, "Row Headers[]"=w304:string[])  [unwired: 1 in]
                    n247 = property class="Tbl"(reference=w306, error in=w303) -> (error out=w302:errorcluster, "Value"=w305:string[][])  [unwired: 1 out]
                    n248 = for {
                      tunnel: w305 -> [w310] mode=indexing
                      tunnel: w304 -> [w311] mode=indexing
                      tunnel: [w308] -> w300 mode=indexing if=w309
                      shift-right: [w307] -> _
                      shift-left: w302 -> [w307]
                      n249 = Build Array (concatenate)(w311, w310) -> (w308:string[])
                      n250 = Index Array(array=w310) -> (element=w312:string)  [unwired: 1 in]
                      n251 = case shown="\"\"" w312 {
                        tunnel: [TRUE FALSE] -> w309
                        frame Default {
                        }
                        frame "" {
                        }
                      }
                    }
                    n252 = global read "追溯Global.vi" "CODEMAIN_ID"() -> (w296:string)
                    n253 = global read "追溯Global.vi" "DEVICE_ID"() -> (w299:string)
                    n254 = global read "追溯Global.vi" "USER_ID"() -> (w298:string)
                    n255 = call "UPRESULT.vi"("DEVICE_ID"=w299, "USER_ID"=w298, "CODE_ID"=w296, "RESULT_VALUE"=w297) -> ()  [unwired: 11 in, 1 out]
                    n256 = call "UPTEST.vi"("Result"=w300, "CODE_ID"=w296, "DEVICE_ID"=w299) -> ()  [unwired: 6 in, 1 out]
                  }
                }
              }
              frame #3 {
                n257 = global read "Global.vi" "传感器码"() -> (w316:string)
                n258 = global read "Global.vi" "产品编号"() -> (w315:string)
                n259 = call "UPCODE.vi"("CODE_SENSOR"=w316, "CODE_MAIN"=w315) -> ()  [unwired: 13 in, 1 out]
              }
              frame #4 {
                n260 = global read "检测结果.vi" "合格状态"() -> (w320:string)
                n261 = local write "STEP"("自动" ("STEP")) -> ()
                n262 = case shown="\"合格\"" w320 {
                  frame "假", Default {
                  }
                  frame "合格" {
                    n263 = global read "Global.vi" "合格数量"() -> (w322:i32)
                    n264 = Increment(x=w322) -> (x+1=w321:i32)
                    n265 = global write "Global.vi" "合格数量"(w321) -> ()
                  }
                }
                n266 = call "备用1.vi"("枚举"=enum16{"Read", "Write"}."Write", "Status_Write"=i16 21) -> ()  [unwired: 9 in, 1 out]
              }
            }
          }
        }
        n267 = global read "Global.vi" "程序关闭"() -> (w10:bool)
      }
    }
  }
